vi "Time since T0.vi"(4 "error in (no error)":errorcluster, 6 "T0 millisecond timer value":u32, 7 "Variant (for data flow only)":variant) -> (0 "error out":errorcluster, 2 "Time elapsed (ms)":u32, 3 "current ms":u32)   [LabVIEW 2013]
doc: "This vi measures the time in milliseconds since T0. The variant input is unused. It is provided to establish dataflow with .vi's that do not have error outputs."
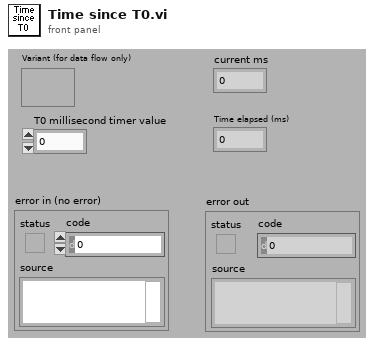
[diagram p1: front panel]
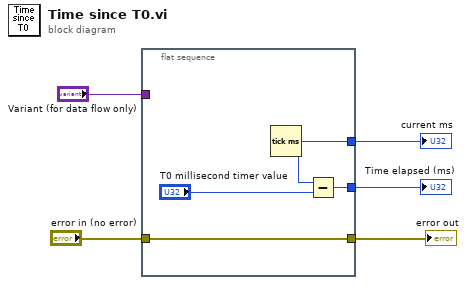
[diagram p0: block diagram]
diagram:
  n1 = flat-sequence {
    tunnel: [w9] -> w5
    tunnel: [w6] -> w4
    tunnel: [w7] -> w3
    tunnel: "error in (no error)" -> [w6]
    tunnel: "Variant (for data flow only)" -> [_]
    frame #0 {
      n2 = Tick Count (ms)() -> (millisecond timer value=w7:u32)
      n3 = Subtract(x=w7, y="T0 millisecond timer value") -> (x-y=w9:u32)
    }
  }
  "Time elapsed (ms)" <- w5
  "error out" <- w4
  "current ms" <- w3
